vi "Mecanum Drive.vi"(6 "Division":dbl=1.0 format="%#_13g", 8 "Turn":dbl format="%#_13g", 9 "Strafe":dbl, 10 "Forward/Backward":dbl, 11 "Mode":enum8{"Start", "Run", "Finish"}(ring)) -> ()   [LabVIEW 2014]
uses:
  <vilib>/Rock Robotics/WPI/RobotDrive/WPI_RobotDriveOpen4MotorWithCANTalonSRX.vi
  <vilib>/Rock Robotics/WPI/RobotDrive/WPI_RobotDriveMecanumDrive_Cartesian.vi
  <vilib>/Rock Robotics/Network Tables/SD Write Numeric Array.vi
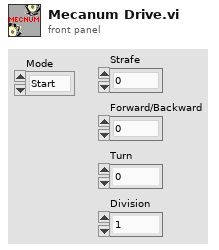
[diagram p1: front panel]
types:
  T1 = typedef "WPI_RobotDriveDevRef.ctl" = cluster{"DevStatus":errorcluster, "Motors[]":T2[], "Square Inputs":bool, "Max Output":dbl}
  T2 = typedef "WPI_MotorControlDeviceRef.ctl" = cluster{"DeviceStatus":errorcluster, "Type":T3, "PWM":cluster{"Controller":T4, "PWM Channel":T5, "DeadBand":T6}, "CAN":cluster{"Device Number":u8, "Control Mode":T7, "Semaphore":T8, "Max Vout":dbl, "TalonSRX Control Mode":T9}, "Invert":bool, "TransformRef":T10, "InvTransformRef":T10}
  T3 = typedef "WPI_MotorControlType.ctl" = enum16{"PWM", "CAN", "CANTalonSRX"}
  T4 = typedef "FPGA_TypedefDigitalModule.ctl" = enum16{"Controller 1"}
  T5 = typedef "FPGA_DIOPWMChannel.ctl" = enum8{"PWM 0", "PWM 1", "PWM 2", "PWM 3", "PWM 4", "PWM 5", "PWM 6", "PWM 7", "PWM 8", "PWM 9", "PWM MXP 0", "PWM MXP 1", "PWM MXP 2", "PWM MXP 3", "PWM MXP 4", "PWM MXP 5", "PWM MXP 6", "PWM MXP 7", "PWM MXP 8", "PWM MXP 9", "Invalid"}
  T6 = typedef "WPI_PWMDeadband.ctl" = cluster{"Name":string, "maxPositivePwm":i32, "minPositivePwm":i32, "centerPwm":i32, "maxNegativePwm":i32, "minNegativePwm":i32, "angularRange":u16}
  T7 = typedef "WPI_CANJaguar_ControlMode.ctl" = enum8{"Percent VBus", "Current", "Speed", "Position", "Voltage"}
  T8 = typedef "Semaphore RefNum" = refnum<k1>
  T9 = typedef "WPI_CANTalonSRX_APIControlMode.ctl" = enum8{"Percent VBus", "Speed", "Position", "Slave", "Unchanged / Invalid"}
  T10 = typedef "WPI_PWMTransform_ConPane.ctl" = refnum<vi>
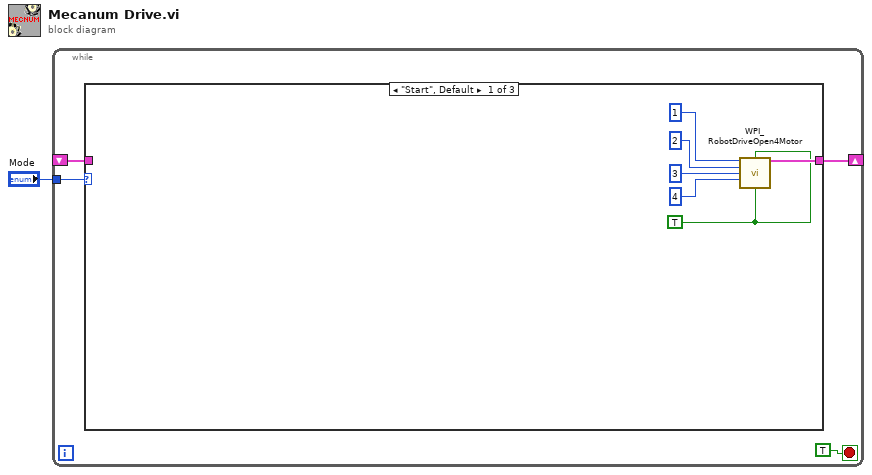
[diagram p0: block diagram]
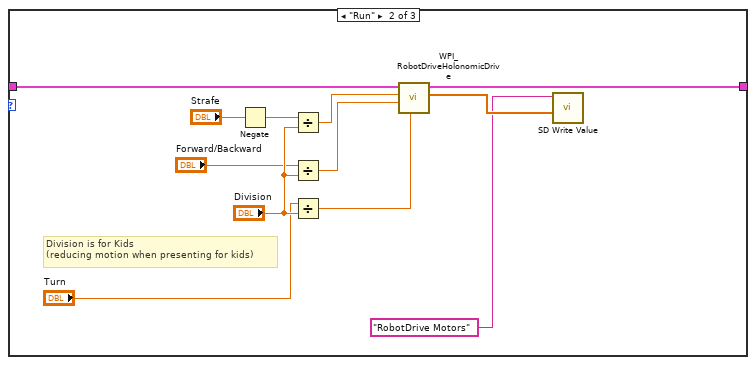
[diagram p2: hidden frame]
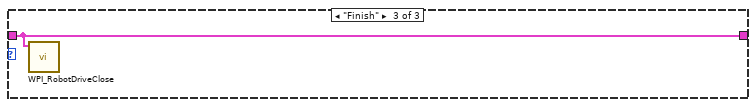
[diagram p3: hidden frame]
diagram:
  n1 = while {
    shift-right: [w5] -> _
    shift-left: _ -> [w4]
    tunnel: "Mode" -> [w3]
    stop <- TRUE stop-if-true
    n2 = case shown="\"Start\", Default" w3 {
      tunnel: [w11 w22 w24] -> w5
      tunnel: w4 -> [_ w23 w24]
      frame "Start", Default {
        w7 = TRUE ("Rear Right Motor Inverted")
        n3 = call-poly <vilib>:"WPI_RobotDriveOpen4Motor.vi"("Rear Left Motor"=u8 1, "Rear Right Motor Inverted"=w7, "Rear Right Motor"=u8 2 ("Rear Left Motor"), "Front Left Motor"=u8 3, "Front Right Motor"=u8 4, "Front Right Motor Inverted"=w7) -> ("RobotDriveDevRef"=w11:T1)  [unwired: 8 in, 1 out]
      }
      frame "Run" {
        # "Division is for Kids\n(reducing motion when presenting for kids)"
        n4 = Negate(x="Strafe") -> (-x=w19:dbl)
        n5 = Divide(x=w19, y="Division") -> (x/y=w21:dbl)
        n6 = Divide(x="Forward/Backward", y="Division") -> (x/y=w14:dbl)
        n7 = Divide(x="Turn", y="Division") -> (x/y=w15:dbl)
        n8 = call-poly <vilib>:"WPI_RobotDriveHolonomicDrive.vi"("Rotation"=w15, "Y"=w14, "X"=w21, "RobotDriveDevRef"=w23) -> ("Motor Values"=w13:dbl[], "RobotDriveDevRef"=w22:T1)  [unwired: 5 in, 1 out]
        n9 = call-poly <vilib>:"SD Write Value.vi"("Numeric Array"=w13, "Name"="RobotDrive Motors") -> ()  [unwired: 8 in, 2 out]
      }
      frame "Finish" {
        n10 = call <vilib>:"WPI_RobotDriveClose.vi"("RobotDriveDevRef"=w24) -> ()  [unwired: 10 in, 1 out]
      }
    }
  }
